vi "SUB_FindSpecificString_NOTrimSpace.vi"(3 "Find this String":string, 5 "String data":string) -> (0 "before \"; \" string":string, 2 "Found":bool)   [LabVIEW 2011]
panel:
  out "after substring":string
  out "match substring":string
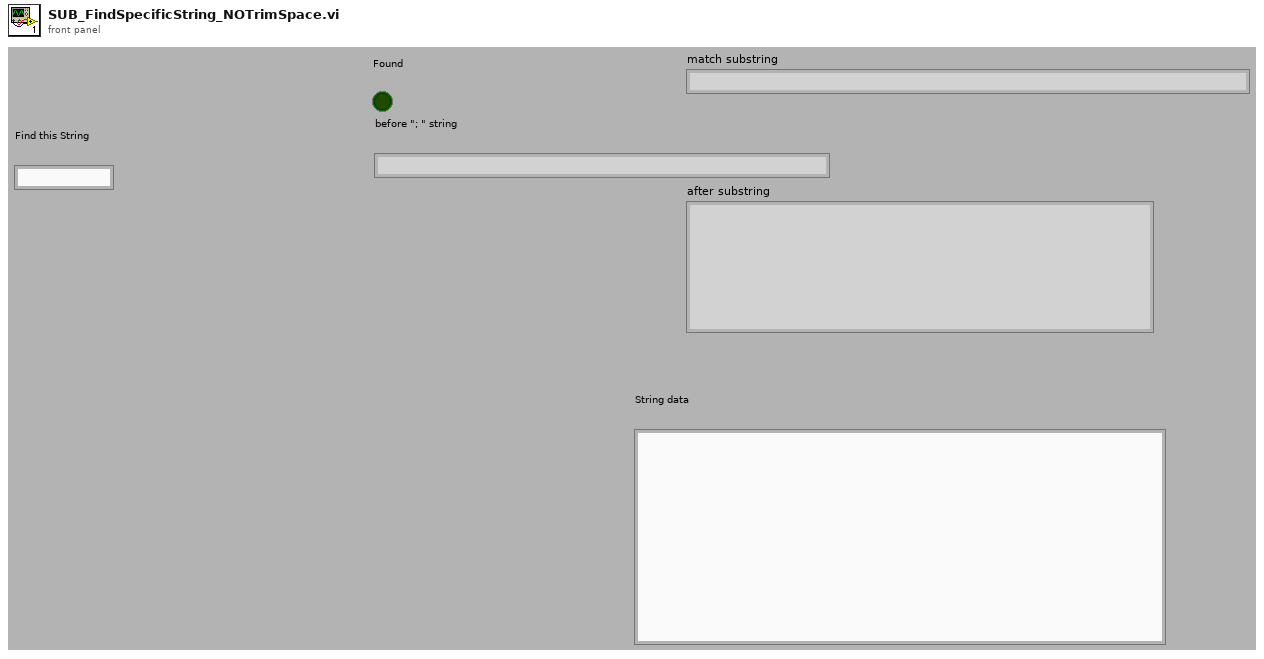
[diagram p1: front panel]
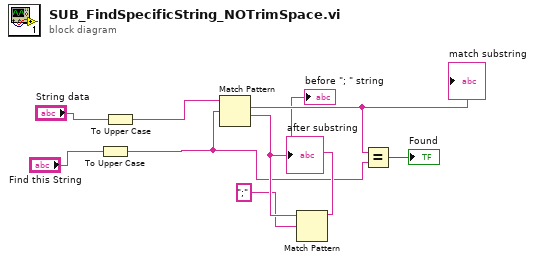
[diagram p0: block diagram]
diagram:
  n1 = To Upper Case(1:"Find this String") -> (0:w1:string)
  n2 = To Upper Case(1:"String data") -> (0:w2:string)
  n3 = Match Pattern(string=w2, regular expression=w1) -> (match substring=w5:string, after substring=w9:string)  [unwired: 1 in, 2 out]
  "match substring" <- w5
  "after substring" <- w9
  n4 = Match Pattern(string=w9, regular expression=";") -> (before substring=→"before \"; \" string":string)  [unwired: 1 in, 3 out]
  n5 = Equal?(x=w5, y=w1) -> (x = y?=→"Found":bool)
